vi "Error - Log.vi"(8 "error in (no error)":errorcluster, 9 "Data":variant, 10 "Error Level":T1, 11 "Error Log Path":path) -> (0 "error out":errorcluster)   [LabVIEW 2017]
doc: "Stores Error Data to external text file.\n[Covers: EH2]"
uses:
  Controls/Error Level.ctl
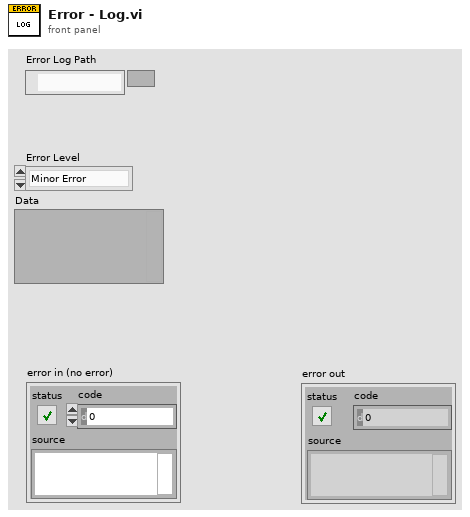
[diagram p1: front panel]
types:
  T1 = typedef "Error Level.ctl" = enum16{"Minor Error", "Wash Cycle Error", "System Error"}
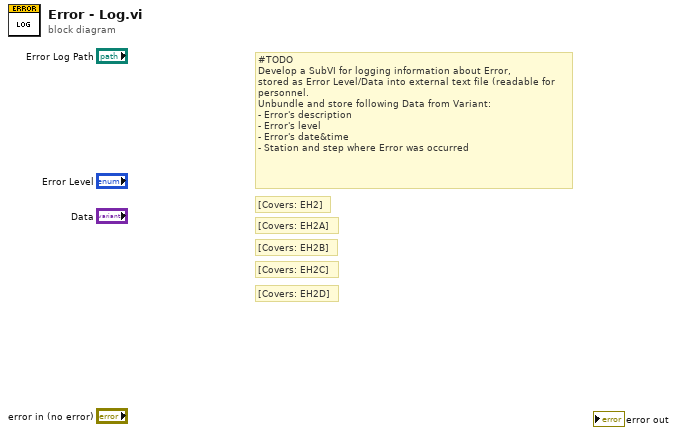
[diagram p0: block diagram]
diagram:
  # "[Covers: EH2D]"
  # "[Covers: EH2C]"
  # "[Covers: EH2B]"
  # "[Covers: EH2A]"
  # "[Covers: EH2]"
  # "#TODO\nDevelop a SubVI for logging information about Error,\nstored as Error Level/Data into external text file (readable for\npersonnel.\nUnbundle and store following Data from Variant:\n- Error's description\n- Error's level\n- Error's date&time\n- Station and step where Error was occurred"
